vi "BRig_RT__Case_Exp__State_setLaserSettings.vi"(6 "input_FPGA_count2ms":dbl, 7 "input_dataExp":u16[](array[numeric]), 9 "input_dataLC":u16[](array[numeric])) -> (10 "output_LR_nTotal_l1":u32, 12 "output_LR_nTotal_l2":u32, 14 "output_LR_reward_nDelay_l1":u32, 15 "output_LR_wrong_nDelay_l1":u32, 16 "output_LR_reward_nDelay_l2":u32, 17 "output_LR_wrong_nDelay_l2":u32)   [LabVIEW 2014]
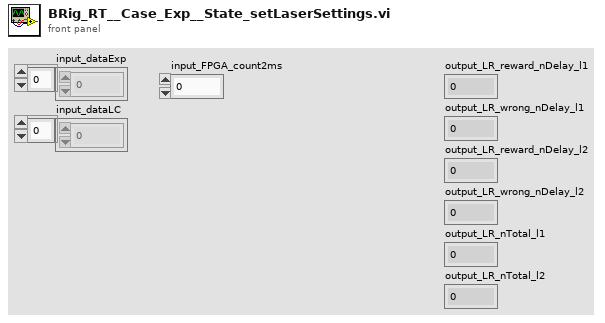
[diagram p1: front panel]
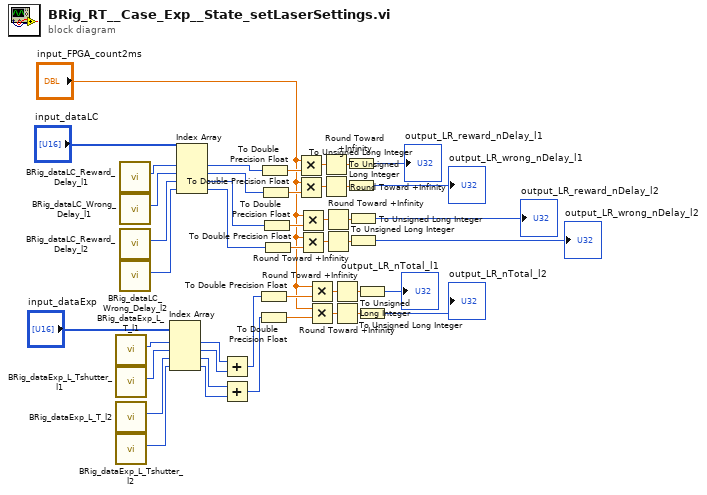
[diagram p0: block diagram]
diagram:
  n1 = call "BRig_dataExp_L_T_l1.vi"() -> ("output_L_T_l1"=w39:i32)  [unwired: 11 in]
  n2 = call "BRig_dataExp_L_Tshutter_l1.vi"() -> ("output_L_Tshutter_l1"=w38:i32)  [unwired: 11 in]
  n3 = call "BRig_dataExp_L_T_l2.vi"() -> ("output_L_T_l2"=w37:i32)  [unwired: 11 in]
  n4 = call "BRig_dataExp_L_Tshutter_l2.vi"() -> ("output_L_Tshutter_l2"=w36:i32)  [unwired: 11 in]
  n5 = call "BRig_dataLC_Reward_Delay_l1.vi"() -> ("output_Reward_Delay"=w23:i32)  [unwired: 11 in]
  n6 = call "BRig_dataLC_Wrong_Delay_l1.vi"() -> ("output_Wrong_Delay"=w20:i32)  [unwired: 11 in]
  n7 = call "BRig_dataLC_Reward_Delay_l2.vi"() -> ("output_Reward_Delay_l2"=w21:i32)  [unwired: 11 in]
  n8 = call "BRig_dataLC_Wrong_Delay_l2.vi"() -> ("output_Wrong_Delay_l2"=w22:i32)  [unwired: 11 in]
  n9 = Index Array(array="input_dataExp", index #1=w39, index #2=w38, index #3=w37, index #4=w36) -> (element #1=w35:u16, element #2=w34:u16, element #3=w33:u16, element #4=w32:u16)
  n10 = Index Array(array="input_dataLC", index #1=w23, index #2=w20, index #3=w21, index #4=w22) -> (element #1=w19:u16, element #2=w18:u16, element #3=w11:u16, element #4=w10:u16)
  n11 = Add(x=w35, y=w34) -> (x+y=w25:u16)
  n12 = Add(x=w33, y=w32) -> (x+y=w24:u16)
  n13 = To Double Precision Float(number=w25) -> (double precision float=w27:dbl)
  n14 = To Double Precision Float(number=w24) -> (double precision float=w26:dbl)
  n15 = To Double Precision Float(number=w19) -> (double precision float=w43:dbl)
  n16 = To Double Precision Float(number=w18) -> (double precision float=w40:dbl)
  n17 = To Double Precision Float(number=w11) -> (double precision float=w15:dbl)
  n18 = To Double Precision Float(number=w10) -> (double precision float=w12:dbl)
  n19 = Multiply(x="input_FPGA_count2ms", y=w43) -> (x*y=w44:dbl)
  n20 = Multiply(x="input_FPGA_count2ms", y=w40) -> (x*y=w41:dbl)
  n21 = Multiply(x="input_FPGA_count2ms", y=w15) -> (x*y=w16:dbl)
  n22 = Multiply(x="input_FPGA_count2ms", y=w12) -> (x*y=w13:dbl)
  n23 = Multiply(x="input_FPGA_count2ms", y=w27) -> (x*y=w29:dbl)
  n24 = Multiply(x="input_FPGA_count2ms", y=w26) -> (x*y=w31:dbl)
  n25 = Round Toward +Infinity(x=w44) -> (ceil(x): smallest int >= x=w45:dbl)
  n26 = Round Toward +Infinity(x=w41) -> (ceil(x): smallest int >= x=w42:dbl)
  n27 = Round Toward +Infinity(x=w16) -> (ceil(x): smallest int >= x=w17:dbl)
  n28 = Round Toward +Infinity(x=w13) -> (ceil(x): smallest int >= x=w14:dbl)
  n29 = Round Toward +Infinity(x=w29) -> (ceil(x): smallest int >= x=w28:dbl)
  n30 = Round Toward +Infinity(x=w31) -> (ceil(x): smallest int >= x=w30:dbl)
  n31 = To Unsigned Long Integer(number=w45) -> (unsigned 32bit integer=→"output_LR_reward_nDelay_l1":u32)
  n32 = To Unsigned Long Integer(number=w42) -> (unsigned 32bit integer=→"output_LR_wrong_nDelay_l1":u32)
  n33 = To Unsigned Long Integer(number=w17) -> (unsigned 32bit integer=→"output_LR_reward_nDelay_l2":u32)
  n34 = To Unsigned Long Integer(number=w14) -> (unsigned 32bit integer=→"output_LR_wrong_nDelay_l2":u32)
  n35 = To Unsigned Long Integer(number=w28) -> (unsigned 32bit integer=→"output_LR_nTotal_l1":u32)
  n36 = To Unsigned Long Integer(number=w30) -> (unsigned 32bit integer=→"output_LR_nTotal_l2":u32)
